vi "PRISM_RasterScan.vi"() -> ()   [LabVIEW 2021]
uses:
  C:/Users/mnopl/Desktop/Software/LabVIEW (deprecated)/PRISM Scanning/Thorlabs.MotionControl.Controls.dll
  LabVIEW (deprecated)/PRISM Scanning/Thorlabs.MotionControl.Controls.dll
  <vilib>/Analysis/baseanly.llb/Mean (DBL).vi
  C:/Users/mnopl/Desktop/Software/LabVIEW (deprecated)/PRISM Scanning/Thorlabs.MotionControl.KCube.StepperMotorCLI.dll
  LabVIEW (deprecated)/PRISM Scanning/Thorlabs.MotionControl.KCube.StepperMotorCLI.dll
  <vilib>/Analysis/NI_AALBase.lvlib
panel:
  in  "Save Image":bool
  in  "Path to save image":path=path "C:/Users/mnopl/Desktop/Data/2022.07.08 - VO2 on TiO2 111/Spectrum_T=RT/Temp.txt"
  in  "Move to cursor":bool
  out "Y origin":dbl=12.636960102246062
  out "X origin":dbl=10.67409113339504
  in  "Auto-level phase":bool
  in  "Acquire":bool=TRUE
  in  "Settle Time Y":u32=1000
  in  "2nd sideband factor":dbl=1.0
  in  "Settle Time X":u32=80
  in  "Py":dbl=-9.096848926680636 format="%_3f"
  in  "Px":dbl=-3.944079495782634 format="%_3f"
  in  "1st sideband offset":dbl
  in  "KCubeStepperControl X":refnum<k24>(container)
  in  "Phase offset":dbl=-1.4748294441662984 format="%_3f"
  out "Phase":dbl[][](graph)
  in  "SerialNumber Z":string="26004283"
  in  "KCubeStepperControl Z":refnum<k24>(container)
  in  "Num Of Steps X":i32=200
  in  "Num Of Steps Y":i32=200
  out "Amplitude":dbl[][](graph)
  in  "Integration time (s)":dbl=0.05
  in  "?":bool
  in  "?":bool
  in  "stop":bool
  in  "Step Size X (um)":sgl=10.0 format="%.8f"
  in  "SerialNumber X":string="26004239"
  in  "Step Size Y (um)":sgl=10.0 format="%.8f"
  in  "SerialNumber Y":string="26004242"
  in  "KCubeStepperControl Y":refnum<k24>(container)
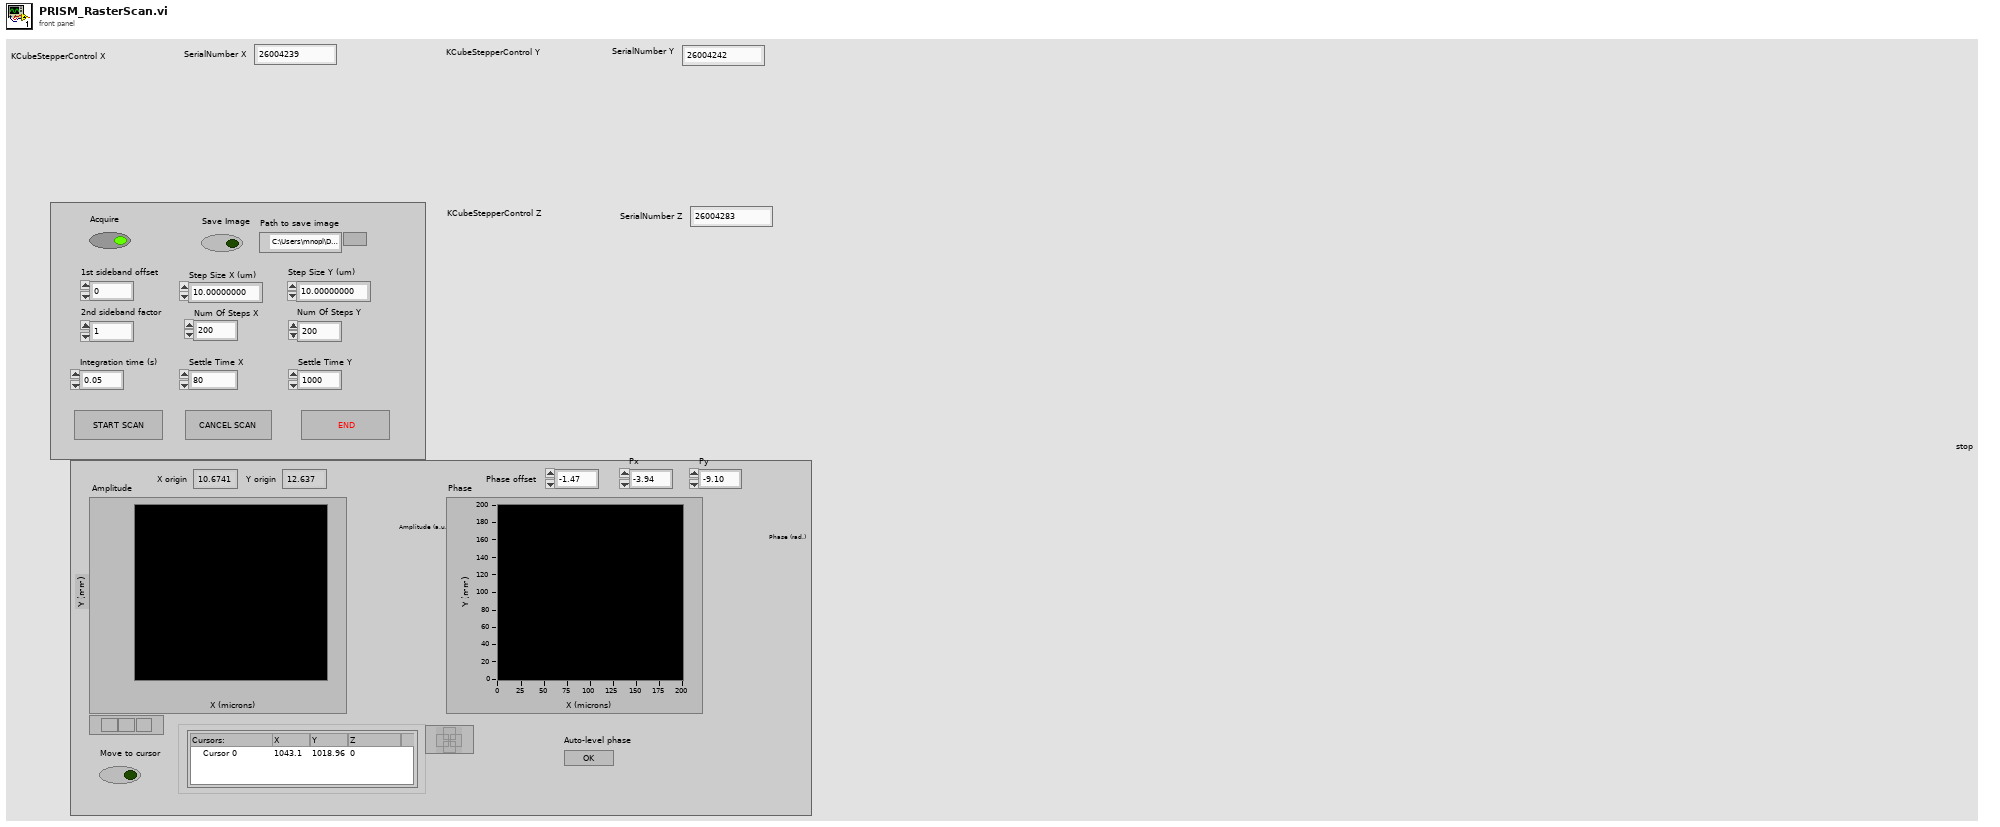
[diagram p1: front panel]
types:
  T1 = typedef "imagedata.ctl" = cluster{"image type":i32, "image depth":i32, "image":u8[], "mask":u8[], "colors":u32[], "Rectangle":cluster{"left":i16, "top":i16, "right":i16, "bottom":i16}}
  T2 = typedef "LVCursorListTypeDef.ctl" = cluster{"Name":string, "Color":u32, "Style":u8, "Point Style":u8, "Name Visible":bool, "Allow Drag":bool, "Cursor Mode":u32, "Plot":i32, "Index":i32, "Position":cluster{"X":dbl, "Y":dbl}, "X Scale":u32, "Y Scale":u32, "Watch Plots":i32[], "Watch All Plots":bool, "Plot Area":i32, "Label Offset":cluster{"X":dbl, "Y":dbl}}[]
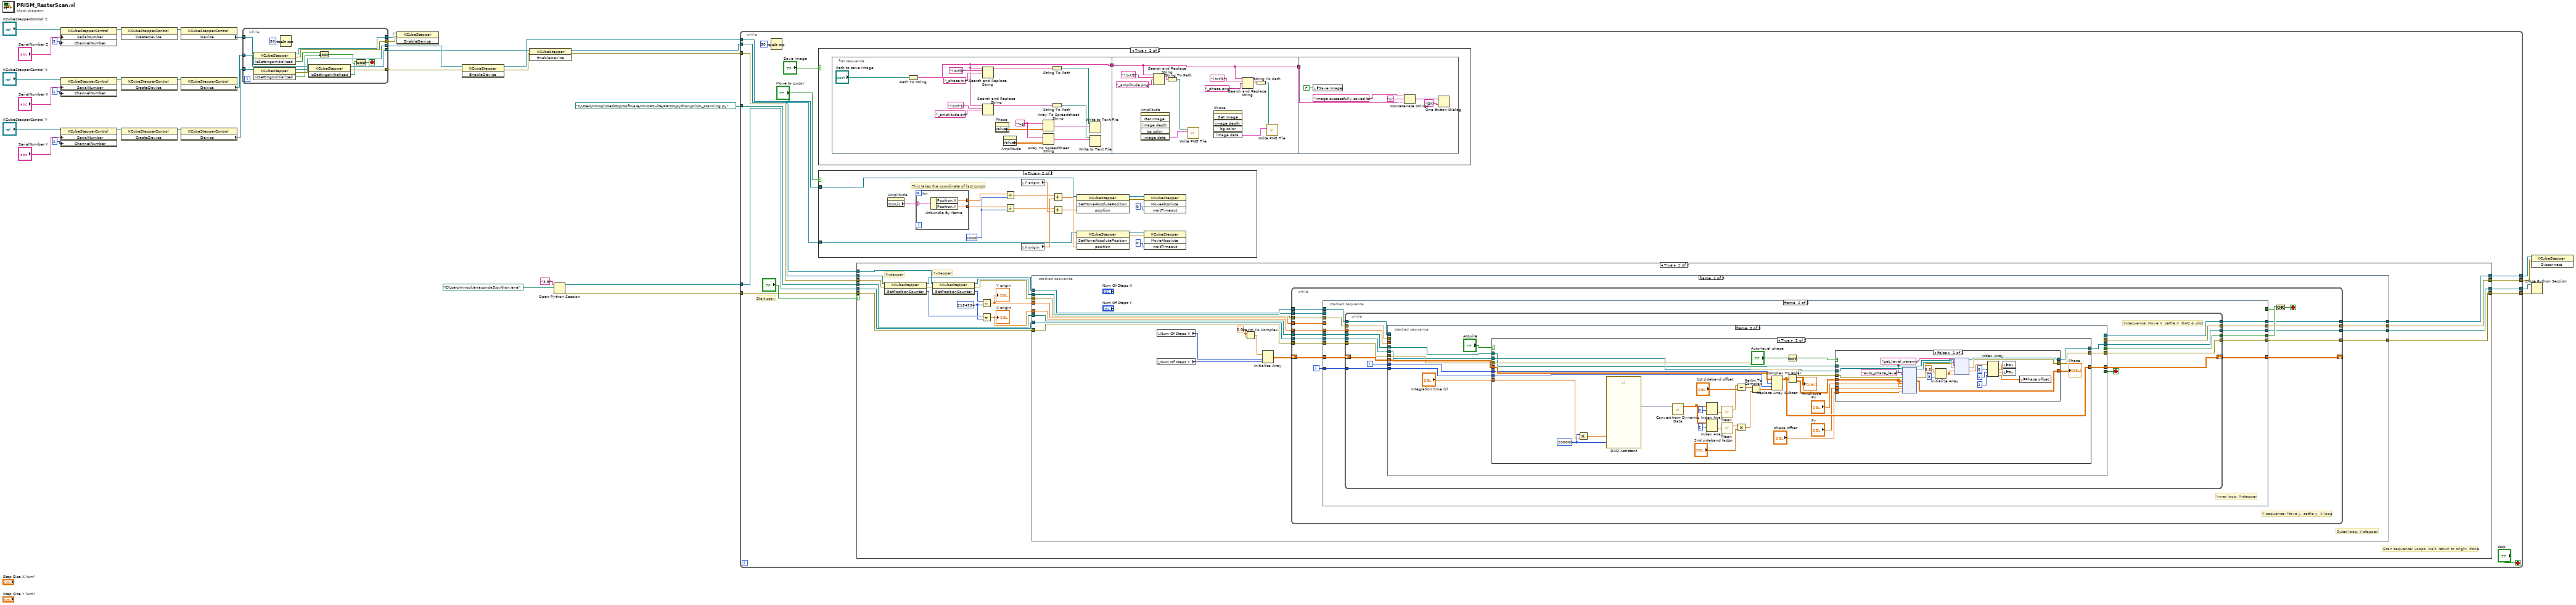
[diagram p0: block diagram]
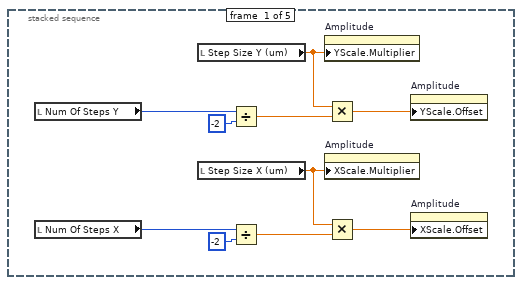
[diagram p5: hidden frame]
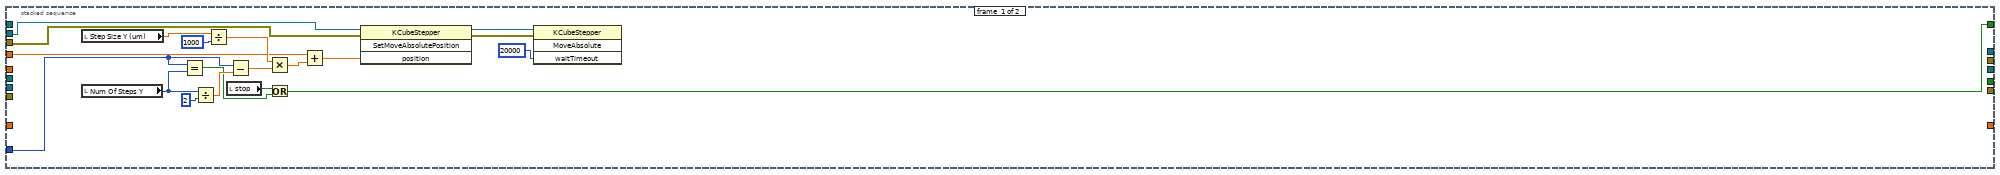
[diagram p6: hidden frame]
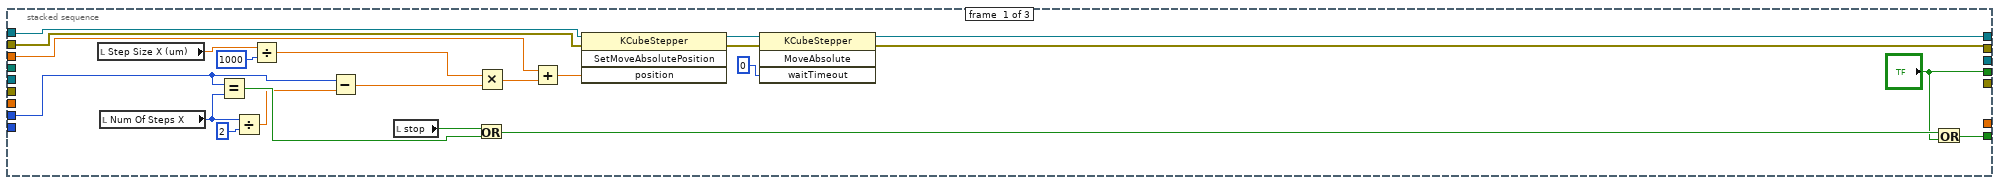
[diagram p7: hidden frame]
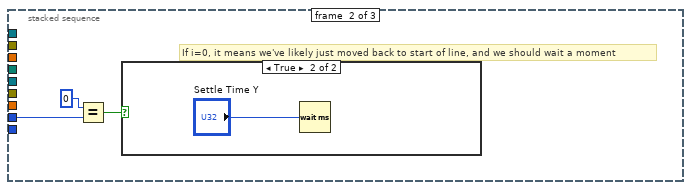
[diagram p8: hidden frame]
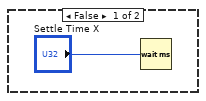
[diagram p9: hidden frame]
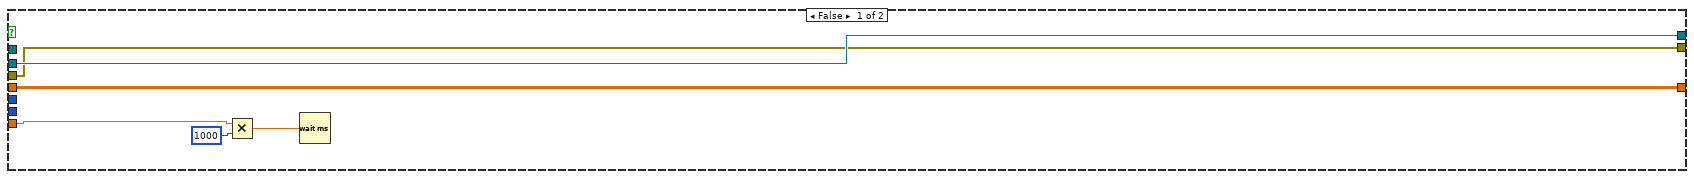
[diagram p10: hidden frame]
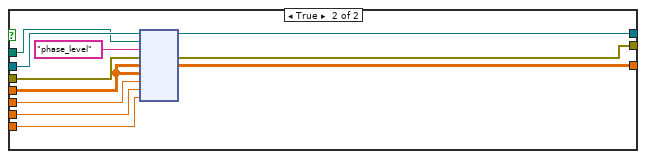
[diagram p11: hidden frame]
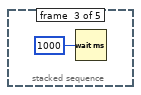
[diagram p12: hidden frame]
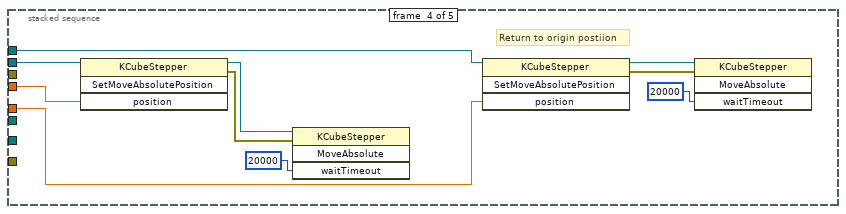
[diagram p13: hidden frame]
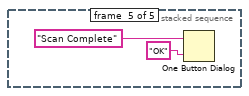
[diagram p14: hidden frame]
diagram:
  n1 = property class="KCubeStepperControl"(reference="KCubeStepperControl Z", "SerialNumber"="SerialNumber Z", "ChannelNumber"=3) -> (reference out=w18:refnum<k24>)  [unwired: 1 in, 1 out]
  n2 = property class="KCubeStepperControl"(reference="KCubeStepperControl X", "SerialNumber"="SerialNumber X", "ChannelNumber"=1) -> (reference out=w32:refnum<k24>)  [unwired: 1 in, 1 out]
  n3 = property class="KCubeStepperControl"(reference="KCubeStepperControl Y", "SerialNumber"="SerialNumber Y", "ChannelNumber"=2) -> (reference out=w35:refnum<k24>)  [unwired: 1 in, 1 out]
  n4 = invoke class="KCubeStepperControl" method="CreateDevice"(reference=w18) -> (reference out=w17:refnum<k24>)  [unwired: 2 in, 2 out]
  n5 = invoke class="KCubeStepperControl" method="CreateDevice"(reference=w32) -> (reference out=w31:refnum<k24>)  [unwired: 2 in, 2 out]
  n6 = invoke class="KCubeStepperControl" method="CreateDevice"(reference=w35) -> (reference out=w34:refnum<k24>)  [unwired: 2 in, 2 out]
  n7 = property class="KCubeStepperControl"(reference=w17) -> ("Device"=w12:refnum<k24>)  [unwired: 1 in, 2 out]
  n8 = property class="KCubeStepperControl"(reference=w31) -> ("Device"=w30:refnum<k24>)  [unwired: 1 in, 2 out]
  n9 = property class="KCubeStepperControl"(reference=w34) -> ("Device"=w10:refnum<k24>)  [unwired: 1 in, 2 out]
  n10 = while {
    tunnel: w10 -> [w50]
    tunnel: w30 -> [w49]
    tunnel: [w46] -> w29
    tunnel: [w39] -> w28
    tunnel: [w45] -> w27
    tunnel: [w40] -> w14
    tunnel: [w41] -> w13
    tunnel: w12 -> [w42]
    stop <- w48 stop-if-true
    n11 = invoke class="KCubeStepper" method="IsSettingsInitialized"(reference=w42) -> (reference out=w40:refnum<k24>, error out=w41:errorcluster, "IsSettingsInitialized"=w37:bool)  [unwired: 2 in]
    n12 = invoke class="KCubeStepper" method="IsSettingsInitialized"(reference=w50) -> (reference out=w39:refnum<k24>, error out=w47:errorcluster, "IsSettingsInitialized"=w38:bool)  [unwired: 2 in]
    n13 = Wait (ms)(milliseconds to wait=u32 50) -> ()  [unwired: 1 out]
    n14 = invoke class="KCubeStepper" method="IsSettingsInitialized"(reference=w49, error in=w47) -> (reference out=w45:refnum<k24>, error out=w46:errorcluster, "IsSettingsInitialized"=w44:bool)  [unwired: 1 in]
    n15 = And(x=w37, y=w38) -> (x .and. y?=w43:bool)
    n16 = And(x=w44, y=w43) -> (x .and. y?=w48:bool)
  }
  n17 = invoke class="KCubeStepper" method="EnableDevice"(reference=w14, error in=w13) -> ()  [unwired: 1 in, 3 out]
  n18 = invoke class="KCubeStepper" method="EnableDevice"(reference=w28, error in=w29) -> (reference out=w22:refnum<k24>, error out=w21:errorcluster)  [unwired: 1 in, 1 out]
  n19 = invoke class="KCubeStepper" method="EnableDevice"(reference=w27, error in=w21) -> (reference out=w20:refnum<k24>, error out=w11:errorcluster)  [unwired: 1 in, 1 out]
  n20 = Open Python Session(python version="3.9", python path=path "C:/Users/mnopl/anaconda3/python.exe") -> (session out=w7:refnum<k35>, error out=w5:errorcluster)  [unwired: 1 in]
  n21 = while {
    tunnel: w22 -> [w53]
    tunnel: w20 -> [w54]
    tunnel: w11 -> [w63]
    tunnel: w7 -> [w62]
    tunnel: path "C:/Users/mnopl/Desktop/Software/mnOPSuite/PRISM/python/prism_scanning.py" -> [w61]
    tunnel: w5 -> [w60]
    tunnel: [w59] -> w4
    tunnel: [w58] -> w3
    tunnel: [w57] -> w2
    tunnel: [w56] -> w1
    stop <- "stop" stop-if-true
    # "Start scan"
    n22 = Wait (ms)(milliseconds to wait=50) -> ()  [unwired: 1 out]
    n23 = case shown="True" "Save Image" {
      frame False {
      }
      frame True {
        n24 = flat-sequence {
          tunnel: [w69] -> w68
          tunnel: w68 -> [w84]
          tunnel: [w84] -> w67
          tunnel: w67 -> [w97]
          frame #0 {
            w77 = "%g"
            n25 = Path To String(path="Path to save image") -> (string=w69:string)
            n26 = Search and Replace String(input string=w69, search string="(.txt)$", replace string="_phase.txt") -> (result string=w82:string)  [unwired: 5 in, 3 out]
            n27 = Search and Replace String(input string=w69, search string="(.txt)*$", replace string="_amplitude.txt") -> (result string=w70:string)  [unwired: 5 in, 3 out]
            n28 = property on="Phase" class="IntGraph (strict)"() -> ("Value"=w72:dbl[][])  [unwired: 2 in, 2 out]
            n29 = property on="Amplitude" class="IntGraph (strict)"() -> ("Value"=w71:dbl[][])  [unwired: 2 in, 2 out]
            n30 = Array To Spreadsheet String(array=w72, 3:w77) -> (spreadsheet string=w83:string)  [unwired: 1 in]
            n31 = Array To Spreadsheet String(array=w71, 3:w77) -> (spreadsheet string=w78:string)  [unwired: 1 in]
            n32 = String To Path(string=w82) -> (path=w81:path)
            n33 = String To Path(string=w70) -> (path=w80:path)
            n34 = Write to Text File(file (use dialog)=w81, text=w83) -> ()  [unwired: 2 in, 3 out]
            n35 = Write to Text File(file (use dialog)=w80, text=w78) -> ()  [unwired: 2 in, 3 out]
          }
          frame #1 {
            n36 = invoke on="Amplitude" class="IntGraph (strict)" method="Get Image"() -> ("image data"=w90:T1)  [unwired: 6 in, 5 out]
            n37 = Search and Replace String(input string=w84, search string="(.txt)$", replace string="_amplitude.png") -> (result string=w92:string)  [unwired: 5 in, 3 out]
            n38 = String To Path(string=w92) -> (path=w91:path)
            n39 = call <vilib>:"Write PNG File.vi"("image data"=w90, "path to PNG file"=w91) -> ()  [unwired: 8 in, 2 out]
            n40 = invoke on="Phase" class="IntGraph (strict)" method="Get Image"() -> ("image data"=w86:T1)  [unwired: 6 in, 5 out]
            n41 = Search and Replace String(input string=w84, search string="(.txt)$", replace string="_phase.png") -> (result string=w87:string)  [unwired: 5 in, 3 out]
            n42 = String To Path(string=w87) -> (path=w85:path)
            n43 = call <vilib>:"Write PNG File.vi"("image data"=w86, "path to PNG file"=w85) -> ()  [unwired: 8 in, 2 out]
          }
          frame #2 {
            n44 = local write "Save Image"(FALSE) -> ()
            n45 = Concatenate Strings("Image successfully saved to:" ("message"), "\r", w97) -> (w98:string)
            n46 = One Button Dialog(message=w98, button name ("OK")="OK") -> ()  [unwired: 1 out]
          }
        }
      }
    }
    n47 = case shown="True" "Move to cursor" {
      tunnel: w54 -> [_ w111]
      tunnel: w53 -> [_ w106]
      frame False {
      }
      frame True {
        w103 = 1000
        # "This takes the coordinate of last cursor"
        n48 = property on="Amplitude" class="IntGraph (strict)"() -> ("CrsrLis"=w118:T2)  [unwired: 2 in, 2 out]
        n49 = for {
          tunnel: w118 -> [w121] mode=indexing
          tunnel: [w120] -> w102
          tunnel: [w119] -> w105
          n50 = Unbundle By Name(w121) -> ("Position.X"=w120:dbl, "Position.Y"=w119:dbl)
        }
        n51 = Divide(x=w102, y=w103) -> (x/y=w101:dbl)
        n52 = Divide(x=w105, y=w103) -> (x/y=w104:dbl)
        n53 = local read "Y origin"() -> (w116:dbl)
        n54 = local read "X origin"() -> (w117:dbl)
        n55 = Add(x=w101, y=w117) -> (x+y=w112:dbl)
        n56 = Add(x=w104, y=w116) -> (x+y=w107:dbl)
        n57 = invoke class="KCubeStepper" method="SetMoveAbsolutePosition"(reference=w106, "position"=w107) -> (reference out=w110:refnum<k24>, error out=w109:errorcluster)  [unwired: 2 in, 2 out]
        n58 = invoke class="KCubeStepper" method="SetMoveAbsolutePosition"(reference=w111, "position"=w112) -> (reference out=w115:refnum<k24>, error out=w114:errorcluster)  [unwired: 2 in, 2 out]
        n59 = invoke class="KCubeStepper" method="MoveAbsolute"(reference=w110, error in=w109, "waitTimeout"=0) -> ()  [unwired: 1 in, 4 out]
        n60 = invoke class="KCubeStepper" method="MoveAbsolute"(reference=w115, error in=w114, "waitTimeout"=0) -> ()  [unwired: 1 in, 4 out]
      }
    }
    n61 = case shown="True" "?" {
      tunnel: w54 -> [w123 w141]
      tunnel: w53 -> [_ w143]
      tunnel: w63 -> [w122 w140]
      tunnel: w62 -> [w125 w134]
      tunnel: w61 -> [_ w133]
      tunnel: w60 -> [w124 w132]
      tunnel: [w125 w131] -> w59
      tunnel: [w124 w130] -> w58
      tunnel: [w123 w129] -> w57
      tunnel: [w122 w128] -> w56
      frame False {
      }
      frame True {
        w135 = 2184534
        # "Scan sequence: Loops, wait, return to origin, done"
        # "Y-stepper"
        # "X-stepper"
        n62 = invoke class="KCubeStepper" method="GetPositionCounter"(reference=w141, error in=w140) -> (reference out=w137:refnum<k24>, error out=w139:errorcluster, "GetPositionCounter"=w136:i32)  [unwired: 1 in]
        n63 = invoke class="KCubeStepper" method="GetPositionCounter"(reference=w143, error in=w139) -> (reference out=w142:refnum<k24>, error out=w138:errorcluster, "GetPositionCounter"=w144:i32)  [unwired: 1 in]
        n64 = Divide(x=w144, y=w135) -> (x/y=w126:dbl)
        "Y origin" <- w126
        n65 = Divide(x=w136, y=w135) -> (x/y=w127:dbl)
        "X origin" <- w127
        n66 = stacked-sequence {
          tunnel: w142 -> [_ w159 _ w354 _]
          tunnel: w127 -> [_ w157 _ w355 _]
          tunnel: w137 -> [_ w160 _ w353 _]
          tunnel: w138 -> [_ w161 _ _ _]
          tunnel: w126 -> [_ w158 _ w356 _]
          tunnel: w134 -> [_ w166 _ _ _]
          tunnel: w133 -> [_ w165 _ _ _]
          tunnel: w132 -> [_ w164 _ _ _]
          tunnel: [_ w163 _ _ _] -> w131
          tunnel: [_ w162 _ _ _] -> w130
          tunnel: [_ w156 _ _ _] -> w129
          tunnel: [_ w155 _ _ _] -> w128
          frame #0 {
            n67 = local read "Num Of Steps Y"() -> (w150:i32)
            n68 = local read "Num Of Steps X"() -> (w153:i32)
            n69 = local read "Step Size Y (um)"() -> (w146:sgl)
            n70 = local read "Step Size X (um)"() -> (w148:sgl)
            n71 = Divide(x=w150, y=-2) -> (x/y=w151:dbl)
            n72 = Divide(x=w153, y=-2) -> (x/y=w154:dbl)
            n73 = property on="Amplitude" class="IntGraph (strict)"("YScale.Multiplier"=w146) -> ()  [unwired: 2 in, 2 out]
            n74 = property on="Amplitude" class="IntGraph (strict)"("XScale.Multiplier"=w148) -> ()  [unwired: 2 in, 2 out]
            n75 = Multiply(x=w146, y=w151) -> (x*y=w145:dbl)
            n76 = Multiply(x=w148, y=w154) -> (x*y=w147:dbl)
            n77 = property on="Amplitude" class="IntGraph (strict)"("YScale.Offset"=w145) -> ()  [unwired: 2 in, 2 out]
            n78 = property on="Amplitude" class="IntGraph (strict)"("XScale.Offset"=w147) -> ()  [unwired: 2 in, 2 out]
          }
          frame #1 {
            w168 = 0.0
            # "Outer loop: Y-stepper"
            n79 = local read "Num Of Steps X"() -> (w170:i32)
            n80 = local read "Num Of Steps Y"() -> (w171:i32)
            n81 = Re/Im To Complex(1:w168, 2:w168) -> (0:w167:cdb)
            n82 = Initialize Array(w167, w170, w171) -> (w169:cdb[][])
            n83 = while {
              shift-right: [w186] -> _
              shift-left: w169 -> [w187]
              tunnel: [w185] -> w156
              tunnel: w166 -> [w178]
              tunnel: w165 -> [w173]
              tunnel: w164 -> [w184]
              tunnel: [w183] -> w163
              tunnel: [w182] -> w162
              tunnel: w161 -> [w180]
              tunnel: w160 -> [w177]
              tunnel: w159 -> [w176]
              tunnel: w158 -> [w175]
              tunnel: w157 -> [w174]
              tunnel: [w172] -> w155
              i -> [w179]
              stop <- w188 stop-if-true
              # "Y-sequence: Move y, settle y, X-loop"
              n84 = stacked-sequence {
                tunnel: w187 -> [_ w215]
                tunnel: w184 -> [_ w214]
                tunnel: [_ w222] -> w189
                tunnel: [_ w221] -> w186
                tunnel: [_ w220] -> w185
                tunnel: [_ w219] -> w183
                tunnel: [_ w218] -> w182
                tunnel: [w197 _] -> w181
                tunnel: w180 -> [w193 w217]
                tunnel: w179 -> [w190 w216]
                tunnel: w178 -> [_ w213]
                tunnel: w177 -> [_ w212]
                tunnel: w176 -> [w194 _]
                tunnel: w175 -> [w192 _]
                tunnel: w174 -> [_ w211]
                tunnel: w173 -> [_ w210]
                tunnel: [_ w209] -> w172
                frame #0 {
                  n85 = local read "Step Size Y (um)"() -> (w196:sgl)
                  n86 = local read "Num Of Steps Y"() -> (w202:i32)
                  n87 = Equal?(x=w190, y=w202) -> (x = y?=w200:bool)
                  n88 = Divide(x=w202, y=2) -> (x/y=w206:dbl)
                  n89 = Divide(x=w196, y=1000) -> (x/y=w208:sgl)
                  n90 = local read "stop"() -> (w201:bool)
                  n91 = Subtract(x=w190, y=w206) -> (x-y=w205:dbl)
                  n92 = Multiply(x=w208, y=w205) -> (x*y=w207:dbl)
                  n93 = Or(x=w201, y=w200) -> (x .or. y?=w197:bool)
                  n94 = Add(x=w192, y=w207) -> (x+y=w204:dbl)
                  n95 = invoke class="KCubeStepper" method="SetMoveAbsolutePosition"(reference=w194, error in=w193, "position"=w204) -> (reference out=w195:refnum<k24>, error out=w203:errorcluster)  [unwired: 1 in, 2 out]
                  n96 = invoke class="KCubeStepper" method="MoveAbsolute"(reference=w195, error in=w203, "waitTimeout"=20000) -> ()  [unwired: 1 in, 4 out]
                }
                frame #1 {
                  # "Inner loop: X-stepper"
                  n97 = while {
                    tunnel: w213 -> [w238]
                    tunnel: [w237] -> w220
                    tunnel: [w234] -> w222
                    tunnel: w216 -> [w227]
                    shift-right: [w232] -> w221
                    shift-left: w215 -> [w233]
                    tunnel: w214 -> [w231]
                    tunnel: [w230] -> w219
                    tunnel: [w229] -> w218
                    tunnel: w217 -> [w228]
                    tunnel: w212 -> [w226]
                    tunnel: w211 -> [w225]
                    tunnel: w210 -> [w224]
                    tunnel: [w223] -> w209
                    i -> [w236]
                    stop <- w235 stop-if-true
                    # "X-sequence: Move X, settle X, DAQ & plot"
                    n98 = stacked-sequence {
                      tunnel: w238 -> [_ _ w272]
                      tunnel: [w260 _ _] -> w237
                      tunnel: w228 -> [w259 _ _]
                      tunnel: w236 -> [w251 w263 w270]
                      tunnel: [w253 _ _] -> w235
                      tunnel: ["?" _ _] -> w234
                      tunnel: w233 -> [_ _ w277]
                      tunnel: [_ _ w275] -> w232
                      tunnel: w231 -> [_ _ w276]
                      tunnel: [_ _ w274] -> w230
                      tunnel: [_ _ w273] -> w229
                      tunnel: w227 -> [_ _ w269]
                      tunnel: w226 -> [w242 _ _]
                      tunnel: w225 -> [w241 _ _]
                      tunnel: w224 -> [_ _ w271]
                      tunnel: [w239 _ _] -> w223
                      frame #0 {
                        n99 = local read "Step Size X (um)"() -> (w243:sgl)
                        n100 = local read "Num Of Steps X"() -> (w249:i32)
                        n101 = Equal?(x=w251, y=w249) -> (x = y?=w256:bool)
                        n102 = Divide(x=w249, y=2) -> (x/y=w247:dbl)
                        n103 = Divide(x=w243, y=1000) -> (x/y=w244:sgl)
                        n104 = Subtract(x=w251, y=w247) -> (x-y=w250:dbl)
                        n105 = local read "stop"() -> (w255:bool)
                        n106 = Or(x=w255, y=w256) -> (x .or. y?=w254:bool)
                        n107 = Multiply(x=w244, y=w250) -> (x*y=w246:dbl)
                        n108 = Add(x=w241, y=w246) -> (x+y=w257:dbl)
                        n109 = invoke class="KCubeStepper" method="SetMoveAbsolutePosition"(reference=w242, error in=w259, "position"=w257) -> (reference out=w261:refnum<k24>, error out=w258:errorcluster)  [unwired: 1 in, 2 out]
                        n110 = invoke class="KCubeStepper" method="MoveAbsolute"(reference=w261, error in=w258, "waitTimeout"=0) -> (reference out=w260:refnum<k24>, error out=w239:errorcluster)  [unwired: 1 in, 2 out]
                        n111 = Or(x=w254, y="?") -> (x .or. y?=w253:bool)
                      }
                      frame #1 {
                        # "If i=0, it means we've likely just moved back to start of line, and we should wait a moment"
                        n112 = Equal?(x=0, y=w263) -> (x = y?=w264:bool)
                        n113 = case shown="True" w264 {
                          frame False {
                            n114 = Wait (ms)(milliseconds to wait="Settle Time X") -> ()  [unwired: 1 out]
                          }
                          frame True {
                            n115 = Wait (ms)(milliseconds to wait="Settle Time Y") -> ()  [unwired: 1 out]
                          }
                        }
                      }
                      frame #2 {
                        n116 = case shown="True" "Acquire" {
                          tunnel: w277 -> [w278 w308]
                          tunnel: w276 -> [w279 w304]
                          tunnel: [w278 w301] -> w275
                          tunnel: [w280 w297] -> w274
                          tunnel: [w279 w296] -> w273
                          tunnel: w272 -> [w280 w295]
                          tunnel: w271 -> [_ w294]
                          tunnel: w270 -> [_ w289]
                          tunnel: w269 -> [_ w288]
                          tunnel: "Integration time (s)" -> [w283 w286]
                          frame False {
                            n117 = Multiply(x=w283, y=1000) -> (x*y=w281:dbl)
                            n118 = Wait (ms)(milliseconds to wait=w281) -> ()  [unwired: 1 out]
                          }
                          frame True {
                            w316 = 200000
                            n119 = Multiply(x=w316, y=w286) -> (x*y=w315:dbl)
                            n120 = call "DAQ Assistant"("rate"=w316, "number of samples"=w315) -> ("data"=w314:dynamicdata)  [unwired: 15 in, 2 out]
                            n121 = call "Convert from Dynamic Data"("Dynamic Data Type"=w314) -> ("Array"=w313:dbl[][])  [unwired: 3 in]
                            n122 = Index Array(array=w313, index (row)=0) -> (element=w310:dbl[])  [unwired: 1 in]
                            n123 = Index Array(array=w313, index (row)=1) -> (element=w309:dbl[])  [unwired: 1 in]
                            n124 = call-poly <vilib>:"Mean.vi"("X"=w310) -> ("mean"=w305:dbl)  [unwired: 1 out]
                            n125 = call-poly <vilib>:"Mean.vi"("X"=w309) -> ("mean"=w293:dbl)  [unwired: 1 out]
                            n126 = Subtract(x=w305, y="1st sideband offset") -> (x-y=w287:dbl)
                            n127 = Multiply(x=w293, y="2nd sideband factor") -> (x*y=w292:dbl)
                            n128 = Re/Im To Complex(1:w292, 2:w287) -> (0:w290:cdb)
                            n129 = Replace Array Subset(array=w308, new element=w290, index (row)=w289, index (col)=w288) -> (w301:cdb[][])
                            n130 = Not(x="Auto-level phase") -> (.not. x?=w284:bool)
                            n131 = Complex To Polar(r * e^(i*theta)=w301) -> (r=→"Amplitude":dbl[][], theta=w303:dbl[][])
                            n132 = case shown="False" w284 {
                              tunnel: w304 -> [w338 w350]
                              tunnel: w303 -> [w337 w349]
                              tunnel: [w333 w348] -> w302
                              tunnel: "Phase offset" -> [w334 w347]
                              tunnel: "Px" -> [w336 w346]
                              tunnel: "Py" -> [w335 w345]
                              tunnel: [w331 w344] -> w297
                              tunnel: [w329 w343] -> w296
                              tunnel: w295 -> [w340 w342]
                              tunnel: w294 -> [w328 w341]
                              frame False {
                                n133 = node(w340, w328, "auto_phase_level", w338, w337, w337, w336, w335, w334) -> (w332:refnum<k35>, w330:errorcluster, w333:dbl[][])  [unwired: 4 in, 2 out]
                                n134 = Initialize Array(0.0, 3) -> (w317:dbl[])
                                n135 = node(w332, w328, "get_level_params", w330, w317, w317) -> (w331:refnum<k35>, w329:errorcluster, w323:dbl[])  [unwired: 1 in, 2 out]
                                n136 = Index Array(array=w323, index #1=0, index #2=1, index #3=2) -> (element #1=w326:dbl, element #2=w324:dbl, element #3=w325:dbl)
                                n137 = local write "Px"(w326) -> ()
                                n138 = local write "Py"(w324) -> ()
                                n139 = local write "Phase offset"(w325) -> ()
                              }
                              frame True {
                                n140 = node(w342, w341, "phase_level", w350, w349, w349, w346, w345, w347) -> (w344:refnum<k35>, w343:errorcluster, w348:dbl[][])  [unwired: 4 in, 2 out]
                              }
                            }
                            "Phase" <- w302
                          }
                        }
                      }
                    }
                  }
                }
              }
              n141 = Or(x=w189, y=w181) -> (x .or. y?=w188:bool)
            }
          }
          frame #2 {
            n142 = Wait (ms)(milliseconds to wait=1000) -> ()  [unwired: 1 out]
          }
          frame #3 {
            # "Return to origin postiion"
            n143 = invoke class="KCubeStepper" method="SetMoveAbsolutePosition"(reference=w354, "position"=w356) -> (reference out=w362:refnum<k24>, error out=w360:errorcluster)  [unwired: 2 in, 2 out]
            n144 = invoke class="KCubeStepper" method="MoveAbsolute"(reference=w362, error in=w360, "waitTimeout"=20000) -> ()  [unwired: 1 in, 4 out]
            n145 = invoke class="KCubeStepper" method="SetMoveAbsolutePosition"(reference=w353, "position"=w355) -> (reference out=w359:refnum<k24>, error out=w357:errorcluster)  [unwired: 2 in, 2 out]
            n146 = invoke class="KCubeStepper" method="MoveAbsolute"(reference=w359, error in=w357, "waitTimeout"=20000) -> ()  [unwired: 1 in, 4 out]
          }
          frame #4 {
            n147 = One Button Dialog(message="Scan Complete", button name ("OK")="OK") -> ()  [unwired: 1 out]
          }
        }
      }
    }
  }
  n148 = invoke class="KCubeStepper" method="Disconnect"(reference=w2, error in=w1) -> ()  [unwired: 1 in, 3 out]
  n149 = Close Python Session(session in=w4, error in=w3) -> ()  [unwired: 1 out]
